vi "Peak Detector.vi"(0 "Maximum Width":i16, 1 "PMT to trigger on (0,1,2,3)":u8, 2 "Baselines":i16[](array[numeric])=[0, 0, 0, 0], 8 "Minimum Width":i16, 9 "shifts in":T1={FALSE, "max"=[0, 0, 0, 0], "sum"=[0, 0, 0, 0], "time inside"=0, "time outside"=0, "timeoutside-1"=0}, 10 "Maximum Height":i16, 12 "Minimum Height":i16, 14 "trigger on all":bool, 16 "s1,s2,s3,s4":i16[](array[numeric])=[0, 0, 0, 0]) -> (18 "peak complete?":bool, 19 "shifts out":T1, 24 "peaks data":T2)   [LabVIEW 2009]
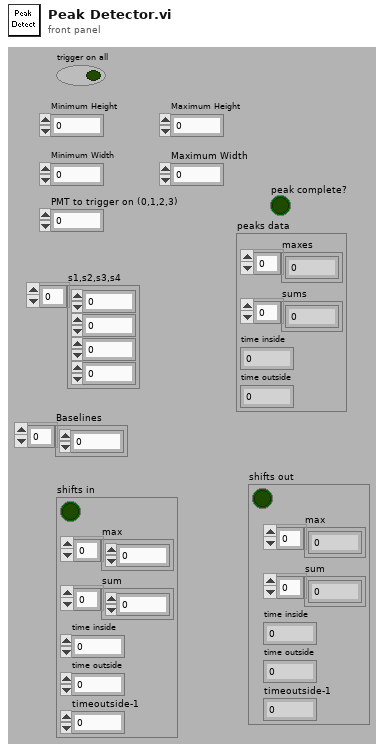
[diagram p1: front panel]
types:
  T1 = cluster{bool, "max":i16[], "sum":i32[], "time inside":i32, "time outside":i32, "timeoutside-1":i32}
  T2 = cluster{"maxes":i16[], "sums":i32[], "time inside":i32, "time outside":i32}
  T3 = cluster{bool, i16[], i32[], i32, i32, "timeoutside-1":i32}
  T4 = cluster{"max":i16[], "sum":i32[], "time inside":i32, "timeoutside-1":i32}
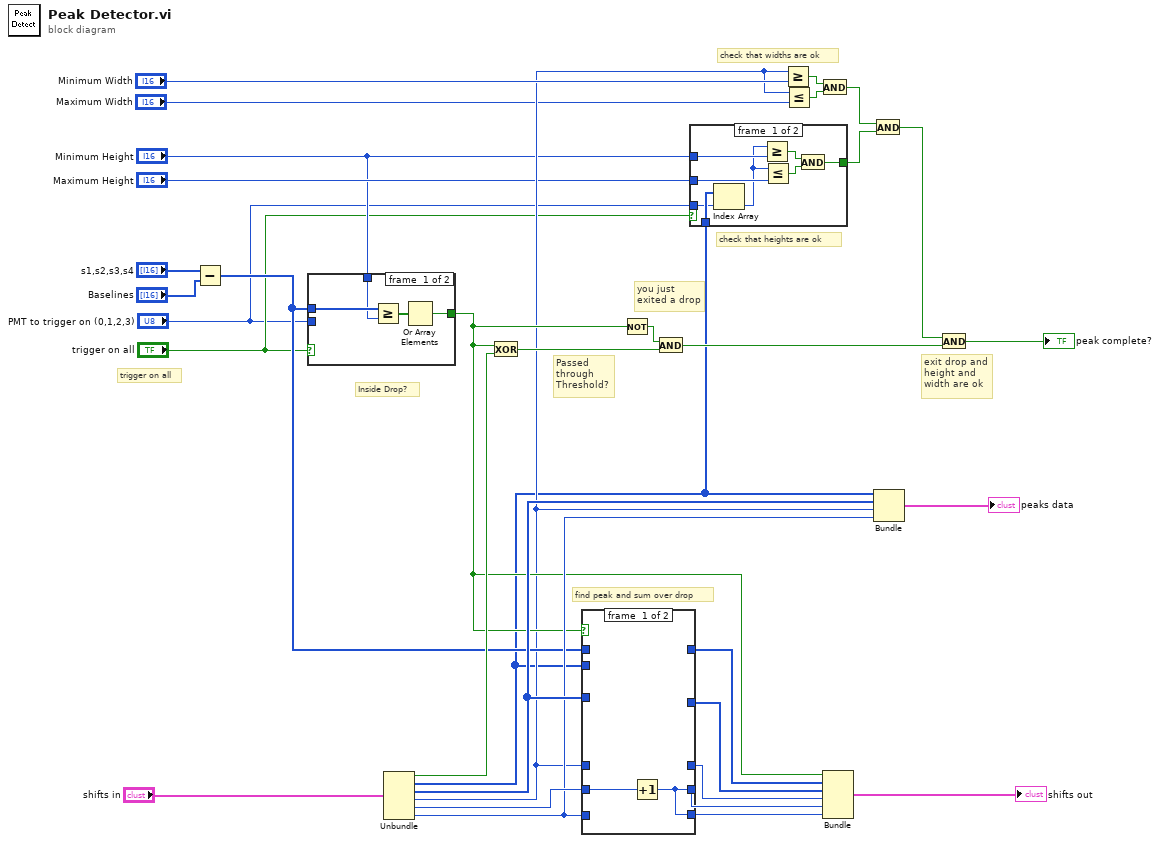
[diagram p0: block diagram]
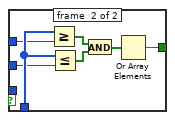
[diagram p2: hidden frame]
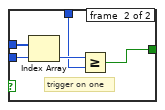
[diagram p3: hidden frame]
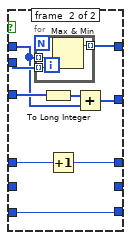
[diagram p4: hidden frame]
diagram:
  # "check that heights are ok"
  # "check that widths are ok"
  # "trigger on all"
  # "Inside Drop?"
  # "find peak and sum over drop"
  # "exit drop and height and width are ok"
  # "you just exited a drop"
  # "Passed through Threshold?"
  n1 = Subtract(x="s1,s2,s3,s4", y="Baselines") -> (x-y=w16:i16[])
  n2 = case shown="False" "trigger on all" {
    tunnel: "Minimum Height" -> [w35 w39]
    tunnel: "PMT to trigger on (0,1,2,3)" -> [_ w42]
    tunnel: [w37 w38] -> w17
    tunnel: w16 -> [w36 w41]
    frame #0 {
      n3 = Greater Or Equal?(x=w36, y=w35) -> (x >= y?=w34:bool[])
      n4 = Or Array Elements(Boolean array=w34) -> (logical OR=w37:bool)
    }
    frame #1 {
      # "trigger on one"
      n5 = Index Array(array=w41, index=w42) -> (element=w40:i16)
      n6 = Greater Or Equal?(x=w40, y=w39) -> (x >= y?=w38:bool)
    }
  }
  n7 = Unbundle("shifts in") -> (w31:bool, "max"=w7:i16[], "sum"=w26:i32[], "time inside"=w11:i32, "time outside"=w22:i32, "timeoutside-1"=w20:i32)
  n8 = Exclusive Or(1:w31, 2:w17) -> (0:w14:bool)
  n9 = case shown="True" w17 {
    tunnel: [_ w51] -> w28
    tunnel: [_ w47] -> w27
    tunnel: w22 -> [w44 _]
    tunnel: [w43 w45] -> w18
    tunnel: w11 -> [_ w46]
    tunnel: [_ w53] -> w32
    tunnel: w16 -> [_ w48]
    tunnel: w26 -> [_ w49]
    tunnel: w7 -> [_ w52]
    tunnel: w20 -> [_ w45]
    tunnel: [w43 _] -> w19
    frame #0 {
      n10 = Increment(x=w44) -> (x+1=w43:i32)
    }
    frame #1 {
      n11 = for {
        tunnel: w52 -> [w56] mode=indexing
        tunnel: [w55] -> w51 mode=indexing
        tunnel: w48 -> [w54] mode=indexing
        n12 = Max & Min(x=w54, y=w56) -> (max(x,y)=w55:i16)  [unwired: 1 out]
      }
      n13 = To Long Integer(number=w49) -> (32bit integer=w50:i32[])
      n14 = Increment(x=w46) -> (x+1=w53:i32)
      n15 = Add(x=w50, y=w48) -> (x+y=w47:i32[])
    }
  }
  n16 = Not(x=w17) -> (.not. x?=w15:bool)
  n17 = And(x=w15, y=w14) -> (x .and. y?=w9:bool)
  n18 = case shown="True" "trigger on all" {
    tunnel: w7 -> [w62 w69]
    tunnel: "Maximum Height" -> [w59 w68]
    tunnel: "Minimum Height" -> [w63 w67]
    tunnel: [w61 w65] -> w3
    tunnel: "PMT to trigger on (0,1,2,3)" -> [w60 _]
    frame #0 {
      n19 = Index Array(array=w62, index=w60) -> (element=w58:i16)
      n20 = Greater Or Equal?(x=w58, y=w63) -> (x >= y?=w64:bool)
      n21 = Less Or Equal?(x=w58, y=w59) -> (x <= y?=w57:bool)
      n22 = And(x=w64, y=w57) -> (x .and. y?=w61:bool)
    }
    frame #1 {
      n23 = Greater Or Equal?(x=w69, y=w67) -> (x >= y?=w71:bool[])
      n24 = Less Or Equal?(x=w69, y=w68) -> (x <= y?=w70:bool[])
      n25 = And(x=w71, y=w70) -> (x .and. y?=w66:bool[])
      n26 = Or Array Elements(Boolean array=w66) -> (logical OR=w65:bool)
    }
  }
  n27 = Greater Or Equal?(x=w11, y="Minimum Width") -> (x >= y?=w12:bool)
  n28 = Less Or Equal?(x=w11, y="Maximum Width") -> (x <= y?=w13:bool)
  n29 = And(x=w12, y=w13) -> (x .and. y?=w4:bool)
  n30 = Bundle(w17, w28, w27, w32, w19, "timeoutside-1"=w18) -> (→"shifts out":T3)  [unwired: 1 in]
  n31 = And(x=w4, y=w3) -> (x .and. y?=w8:bool)
  n32 = Bundle("max"=w7, "sum"=w26, "time inside"=w11, "timeoutside-1"=w20) -> (→"peaks data":T4)  [unwired: 1 in]
  n33 = And(x=w8, y=w9) -> (x .and. y?=→"peak complete?":bool)
